vi "Asset Utilization Example.vi"() -> ()   [LabVIEW 2020]
uses:
  <vilib>/Skyline/Configuration/Configuration HTTP_class/NI Skyline Configuration HTTP.lvclass/NI Skyline Configuration HTTP.ctl
  <vilib>/Skyline/Configuration/Configuration HTTP_class/Open Configuration HTTP.vi
  <vilib>/Skyline/Configuration/HTTP/Open Configuration (Desktop).vi
  <vilib>/Skyline/Configuration/Configuration HTTP_class/NI Skyline Configuration HTTP.lvclass
  <vilib>/Skyline/Configuration/Configuration_class/NI Skyline Configuration.lvclass
panel:
  out "Collecting Past Asset Data":i32(slide) scale=0.0..1000.0
  out "Collecting Asset Data":i32(slide) scale=0.0..591.0
  in  "Password":string
  in  "Username":string="admin"
  in  "Server":string="https://localhost"
  out "Past Asset Utilization":string[][](table)
  out "Assets In Use":string[][](table)
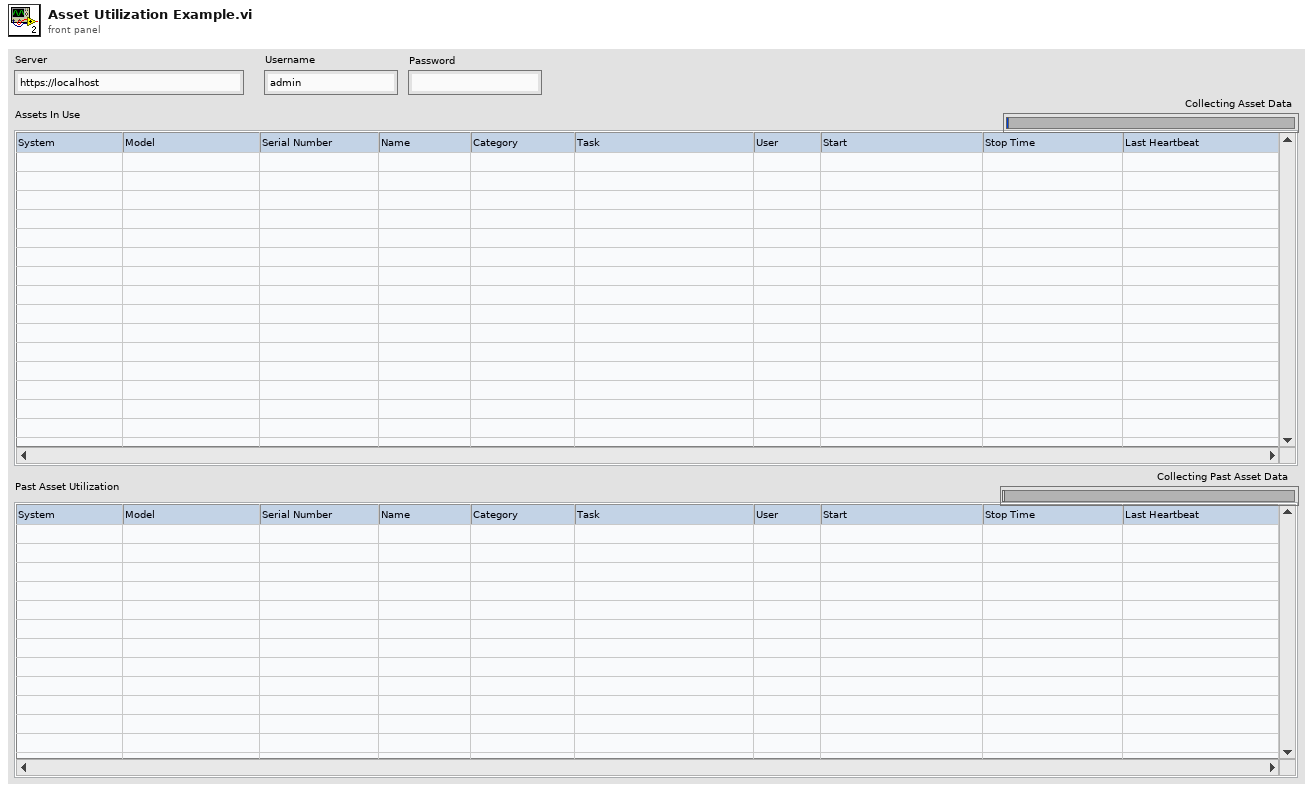
[diagram p1: front panel]
types:
  T1 = cluster{"utilizationIdentifier":string, "assetIdentifier":string, "minionId":string, "category":string, "taskName":string, "userName":string, "startTimestamp":string, "endTimestamp":string, "heartbeatTimestamp":string}[]
  T2 = cluster{"modelName":string, "serialNumber":string, "vendorName":string, "name":string, "location":cluster{"systemName":string}}
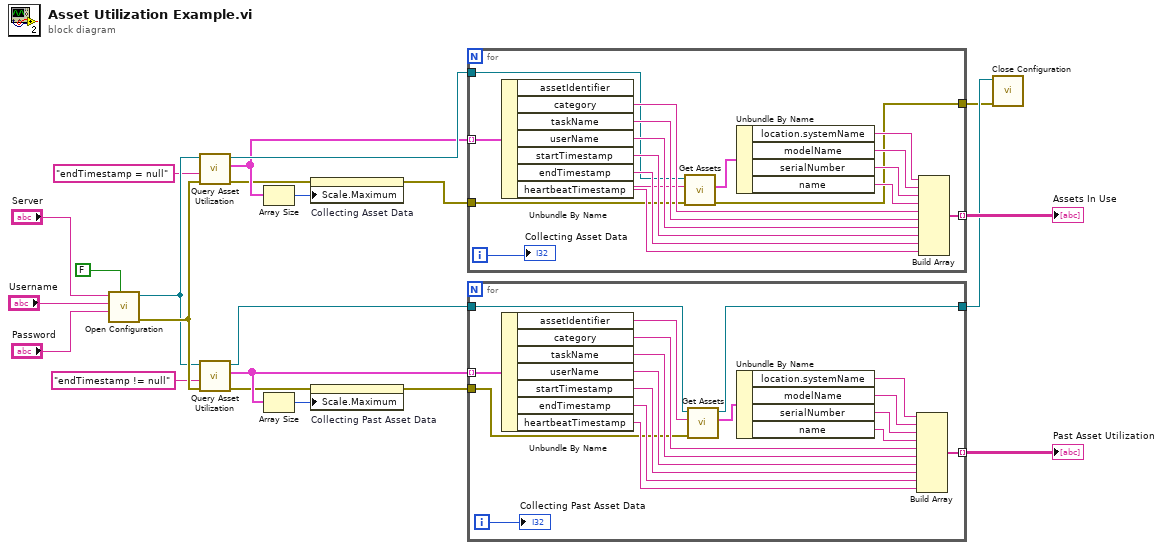
[diagram p0: block diagram]
diagram:
  n1 = call-poly <vilib>:"Open Configuration.vi"("verify server?"=FALSE, "password"="Password", "username"="Username", "server url"="Server") -> ("error out"=w18:errorcluster, "configuration"=w17:refnum<class "NI Skyline Configuration HTTP.lvclass">)  [unwired: 6 in]
  n2 = call "Query Asset Utilization.vi"("Error In"=w18, "Utilization Filter"="endTimestamp = null", "Session In"=w17) -> ("Error Out"=w3:errorcluster, "Asset Utilization"=w8:T1, "Session Out"=w20:refnum<class "NI Skyline Configuration HTTP.lvclass">)  [unwired: 6 in]
  n3 = call "Query Asset Utilization.vi"("Error In"=w18, "Utilization Filter"="endTimestamp != null" ("Asset Filter"), "Session In"=w17) -> ("Error Out"=w5:errorcluster, "Asset Utilization"=w7:T1, "Session Out"=w19:refnum<class "NI Skyline Configuration HTTP.lvclass">)  [unwired: 6 in]
  n4 = Array Size(array=w8) -> (size(s)=w1:i32)
  n5 = Array Size(array=w7) -> (size(s)=w6:i32)
  n6 = property on="Collecting Asset Data" class="Slide (strict)"(error in=w3, "Scale.Maximum"=w1) -> (error out=w2:errorcluster)  [unwired: 1 in, 1 out]
  n7 = property on="Collecting Past Asset Data" class="Slide (strict)"(error in=w5, "Scale.Maximum"=w6) -> (error out=w4:errorcluster)  [unwired: 1 in, 1 out]
  n8 = for {
    tunnel: w8 -> [w40] mode=indexing
    tunnel: [w33] -> w22 mode=indexing
    tunnel: w20 -> [w32]
    tunnel: w2 -> [w31]
    tunnel: [w24] -> w9
    i -> [w23]
    n9 = Unbundle By Name(w40) -> ("assetIdentifier"=w25:string, "category"=w39:string, "taskName"=w38:string, "userName"=w37:string, "startTimestamp"=w36:string, "endTimestamp"=w35:string, "heartbeatTimestamp"=w34:string)
    n10 = call "Get Assets.vi"("Error In"=w31, "Asset ID"=w25, "Session In"=w32) -> ("Error Out"=w24:errorcluster, "Asset"=w26:T2)  [unwired: 6 in, 1 out]
    n11 = Unbundle By Name(w26) -> ("location.systemName"=w30:string, "modelName"=w29:string, "serialNumber"=w28:string, "name"=w27:string)
    n12 = Build Array(w30, w29, w28, w27, w39, w38, w37, w36, w35, w34) -> (w33:string[])
    "Collecting Asset Data" <- w23
  }
  "Assets In Use" <- w22
  n13 = for {
    tunnel: w7 -> [w58] mode=indexing
    tunnel: [w51] -> w16 mode=indexing
    tunnel: w19 -> [w50]
    tunnel: w4 -> [w49]
    tunnel: [w42] -> w10
    i -> [w41]
    n14 = Unbundle By Name(w58) -> ("assetIdentifier"=w43:string, "category"=w57:string, "taskName"=w56:string, "userName"=w55:string, "startTimestamp"=w54:string, "endTimestamp"=w53:string, "heartbeatTimestamp"=w52:string)
    n15 = call "Get Assets.vi"("Error In"=w49, "Asset ID"=w43, "Session In"=w50) -> ("Asset"=w44:T2, "Session Out"=w42:refnum<class "NI Skyline Configuration HTTP.lvclass">)  [unwired: 6 in, 1 out]
    n16 = Unbundle By Name(w44) -> ("location.systemName"=w48:string, "modelName"=w47:string, "serialNumber"=w46:string, "name"=w45:string)
    n17 = Build Array(w48, w47, w46, w45, w57, w56, w55, w54, w53, w52) -> (w51:string[])
    "Collecting Past Asset Data" <- w41
  }
  "Past Asset Utilization" <- w16
  n18 = call-dynamic "Close Configuration.vi"("error in (no error)"=w9, "configuration"=w10) -> ()  [unwired: 9 in, 1 out]
